vi "achat_MP.vi"   [LabVIEW 2024]
uses:
  Prix_MP.vi
  Stock_MP.vi
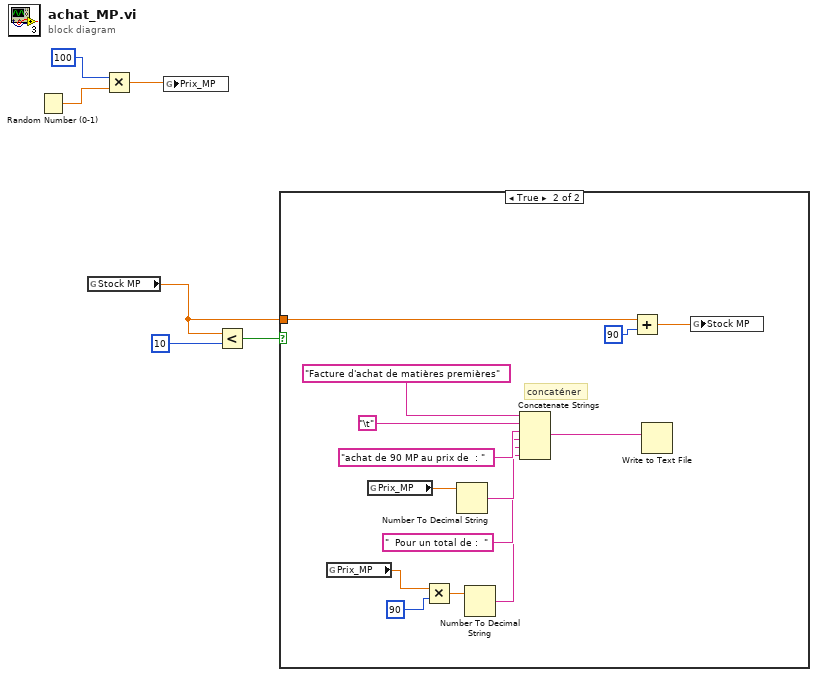
[diagram p0: block diagram]
diagram:
  n1 = Random Number (0-1)() -> (number: 0 to 1=w3:dbl)
  n2 = global read "Stock_MP.vi" "Stock MP"() -> (w2:dbl)
  n3 = Multiply(x=100, y=w3) -> (x*y=w1:dbl)
  n4 = global write "Prix_MP.vi" "Prix_MP"(w1) -> ()
  n5 = Less?(x=w2, y=10) -> (x < y?=w5:bool)
  n6 = case shown="True" w5 {
    tunnel: w2 -> [_ w19]
    frame False {
    }
    frame True {
      # "concaténer"
      n7 = global read "Prix_MP.vi" "Prix_MP"() -> (w8:dbl)
      n8 = global read "Prix_MP.vi" "Prix_MP"() -> (w7:dbl)
      n9 = Multiply(x=w8, y=90) -> (x*y=w11:dbl)
      n10 = Number To Decimal String(number=w7) -> (decimal integer string=w14:string)  [unwired: 1 in]
      n11 = Number To Decimal String(number=w11) -> (decimal integer string=w10:string)  [unwired: 1 in]
      n12 = Concatenate Strings("Facture d'achat de matières premières" ("chaîne"), "\t", "achat de 90 MP au prix de  : ", w14, "  Pour un total de :  ", w10) -> (w9:string)
      n13 = Add(x=w19, y=90) -> (x+y=w18:dbl)
      n14 = Write to Text File(text=w9) -> ()  [unwired: 3 in, 3 out]
      n15 = global write "Stock_MP.vi" "Stock MP"(w18) -> ()
    }
  }
